vi "ZeroMQ Command Generator.vi"() -> ()   [LabVIEW 2018]
uses:
  <vilib>/addons/zeromq/socket_type.ctl
  <vilib>/addons/zeromq/socket_options.ctl
  <vilib>/addons/zeromq/zmq_context.lvclass
  <vilib>/addons/zeromq/zeromq.lvlib
  <vilib>/addons/zeromq/zmq_socket.lvclass
panel:
  out "reply":string
  in  "data":string="hello"
  in  "send":bool
  in  "reqEndpoint":string="tcp://200.131.64.126:54883"
  out "repMsg":string
  in  "repEndpoint":string="tcp://200.131.64.126:54032"
  in  "appendCR":bool caption="Append \n CR-LF"
  in  "pushAddress":string="tcp://200.131.64.170:54031" caption="PUSH address (=PUB+1, before start)"
  out "ledFocuser":bool
  out "ledWeather":bool
  out "ledTCSPD":bool
  out "ledS4ICS":bool
  in  "0mqPubAarray":string[](array[string])=["tcp://200.131.64.237:7001", "tcp://200.131.64.237:7005", "tcp://200.131.64.236:50350", "tcp://200.131.64.126:54030"] caption="Publisher Addresses"
  out "dataS4ICS":string caption="S4ICS"
  in  "stop":bool
  in  "push":bool caption="PUSH"
  in  "cmd in":string="{ \"clientId\": 666,  \"clientTransactionId\": 0,\n        \"clientName\": \"Simulator\", \"action\": \"STATUS\" }" caption="Message to send"
  out "dataFocuser":string caption="Focuser 160"
  out "dataMeteor":string caption="Estação Meteorológica"
  out "dataTCSPD":string caption="TCSPD"
  # "ZeroMQ Command Simulator - SUB & PUSH"
  # "Pedido de status para WheatherT160:"
  # "{ \"clientId\": 123, \"clientTransactionId\": 1234, \"clientName\": \"Simulator\", \"action\": \"STATUS\" }"
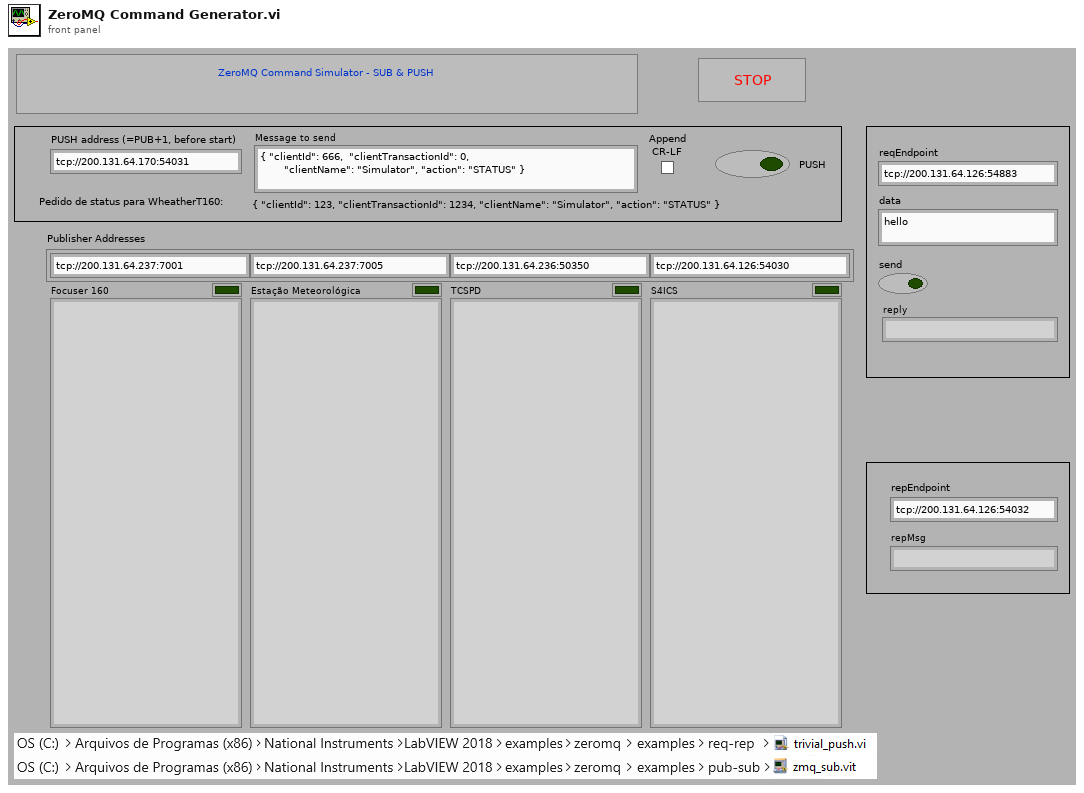
[diagram p1: front panel]
types:
  T1 = typedef "zeromq.lvlib/socket_type.ctl" = enum8{"ZMQ_PAIR", "ZMQ_PUB", "ZMQ_SUB", "ZMQ_REQ", "ZMQ_REP", "ZMQ_DEALER", "ZMQ_ROUTER", "ZMQ_PULL", "ZMQ_PUSH", "ZMQ_XPUB", "ZMQ_XSUB", "ZMQ_STREAM", "ZMQ_SERVER", "ZMQ_CLIENT", "ZMQ_RADIO", "ZMQ_DISH", "ZMQ_GATHER", "ZMQ_SCATTER", "ZMQ_DGRAM"}
  T2 = typedef "zeromq.lvlib/socket_options.ctl" = enum8{"NONE", "ZMQ_HWM", "<2>", "ZMQ_SWAP", "ZMQ_AFFINITY", "ZMQ_ROUTING_ID", "ZMQ_SUBSCRIBE", "ZMQ_UNSUBSCRIBE", "ZMQ_RATE", "ZMQ_RECOVERY_IVL", "ZMQ_MCAST_LOOP", "ZMQ_SNDBUF", "ZMQ_RCVBUF", "ZMQ_RCVMORE", "ZMQ_FD", "ZMQ_EVENTS", "ZMQ_TYPE", "ZMQ_LINGER", "ZMQ_RECONNECT_IVL", "ZMQ_BACKLOG", "ZMQ_RECOVERY_IVL_MSEC", "ZMQ_RECONNECT_IVL_MAX", "ZMQ_MAXMSGSIZE", "ZMQ_SNDHWM", "ZMQ_RCVHWM", "ZMQ_MULTICAST_HOPS", "<26>", "ZMQ_RCVTIMEO", "ZMQ_SNDTIMEO", "<29>", "<30>", "ZMQ_IPV4ONLY", "ZMQ_LAST_ENDPOINT", "ZMQ_ROUTER_MANDATORY", "ZMQ_TCP_KEEPALIVE", "ZMQ_TCP_KEEPALIVE_CNT", "ZMQ_TCP_KEEPALIVE_IDLE", "ZMQ_TCP_KEEPALIVE_INTVL", "ZMQ_TCP_ACCEPT_FILTER", "ZMQ_IMMEDIATE", "ZMQ_XPUB_VERBOSE", "ZMQ_ROUTER_RAW", "ZMQ_IPV6", "ZMQ_MECHANISM", "ZMQ_PLAIN_SERVER", "ZMQ_PLAIN_USERNAME", "ZMQ_PLAIN_PASSWORD", "ZMQ_CURVE_SERVER", "ZMQ_CURVE_PUBLICKEY", "ZMQ_CURVE_SECRETKEY", "ZMQ_CURVE_SERVERKEY", "ZMQ_PROBE_ROUTER", "ZMQ_REQ_CORRELATE", "ZMQ_REQ_RELAXED", "ZMQ_CONFLATE", "ZMQ_ZAP_DOMAIN", "ZMQ_ROUTER_HANDOVER", "ZMQ_TOS", "ZMQ_IPC_FILTER_PID", "ZMQ_IPC_FILTER_UID", "ZMQ_IPC_FILTER_GID", "ZMQ_CONNECT_ROUTING_ID", "ZMQ_GSSAPI_SERVER", "ZMQ_GSSAPI_PRINCIPAL", "ZMQ_GSSAPI_SERVICE_PRINCIPAL", "ZMQ_GSSAPI_PLAINTEXT", "ZMQ_HANDSHAKE_IVL", "<67>", "ZMQ_SOCKS_PROXY", "ZMQ_XPUB_NODROP", "ZMQ_BLOCKY", "ZMQ_XPUB_MANUAL", "ZMQ_XPUB_WELCOME_MSG", "ZMQ_STREAM_NOTIFY", "ZMQ_INVERT_MATCHING", "ZMQ_HEARTBEAT_IVL", "ZMQ_HEARTBEAT_TTL", "ZMQ_HEARTBEAT_TIMEOUT", "ZMQ_XPUB_VERBOSER", "ZMQ_CONNECT_TIMEOUT", "ZMQ_TCP_MAXRT", "ZMQ_THREAD_SAFE", "<82>", "<83>", "ZMQ_MULTICAST_MAXTPDU", "ZMQ_VMCI_BUFFER_SIZE", "ZMQ_VMCI_BUFFER_MIN_SIZE", "ZMQ_VMCI_BUFFER_MAX_SIZE", "ZMQ_VMCI_CONNECT_TIMEOUT", "ZMQ_USE_FD", "ZMQ_GSSAPI_PRINCIPAL_NAMETYPE", "ZMQ_GSSAPI_SERVICE_PRINCIPAL_NAMETYPE", "ZMQ_BINDTODEVICE", "ZMQ_ZAP_ENFORCE_DOMAIN", "ZMQ_LOOPBACK_FASTPATH", "ZMQ_METADATA", "ZMQ_MULTICAST_LOOP", "ZMQ_ROUTER_NOTIFY"}
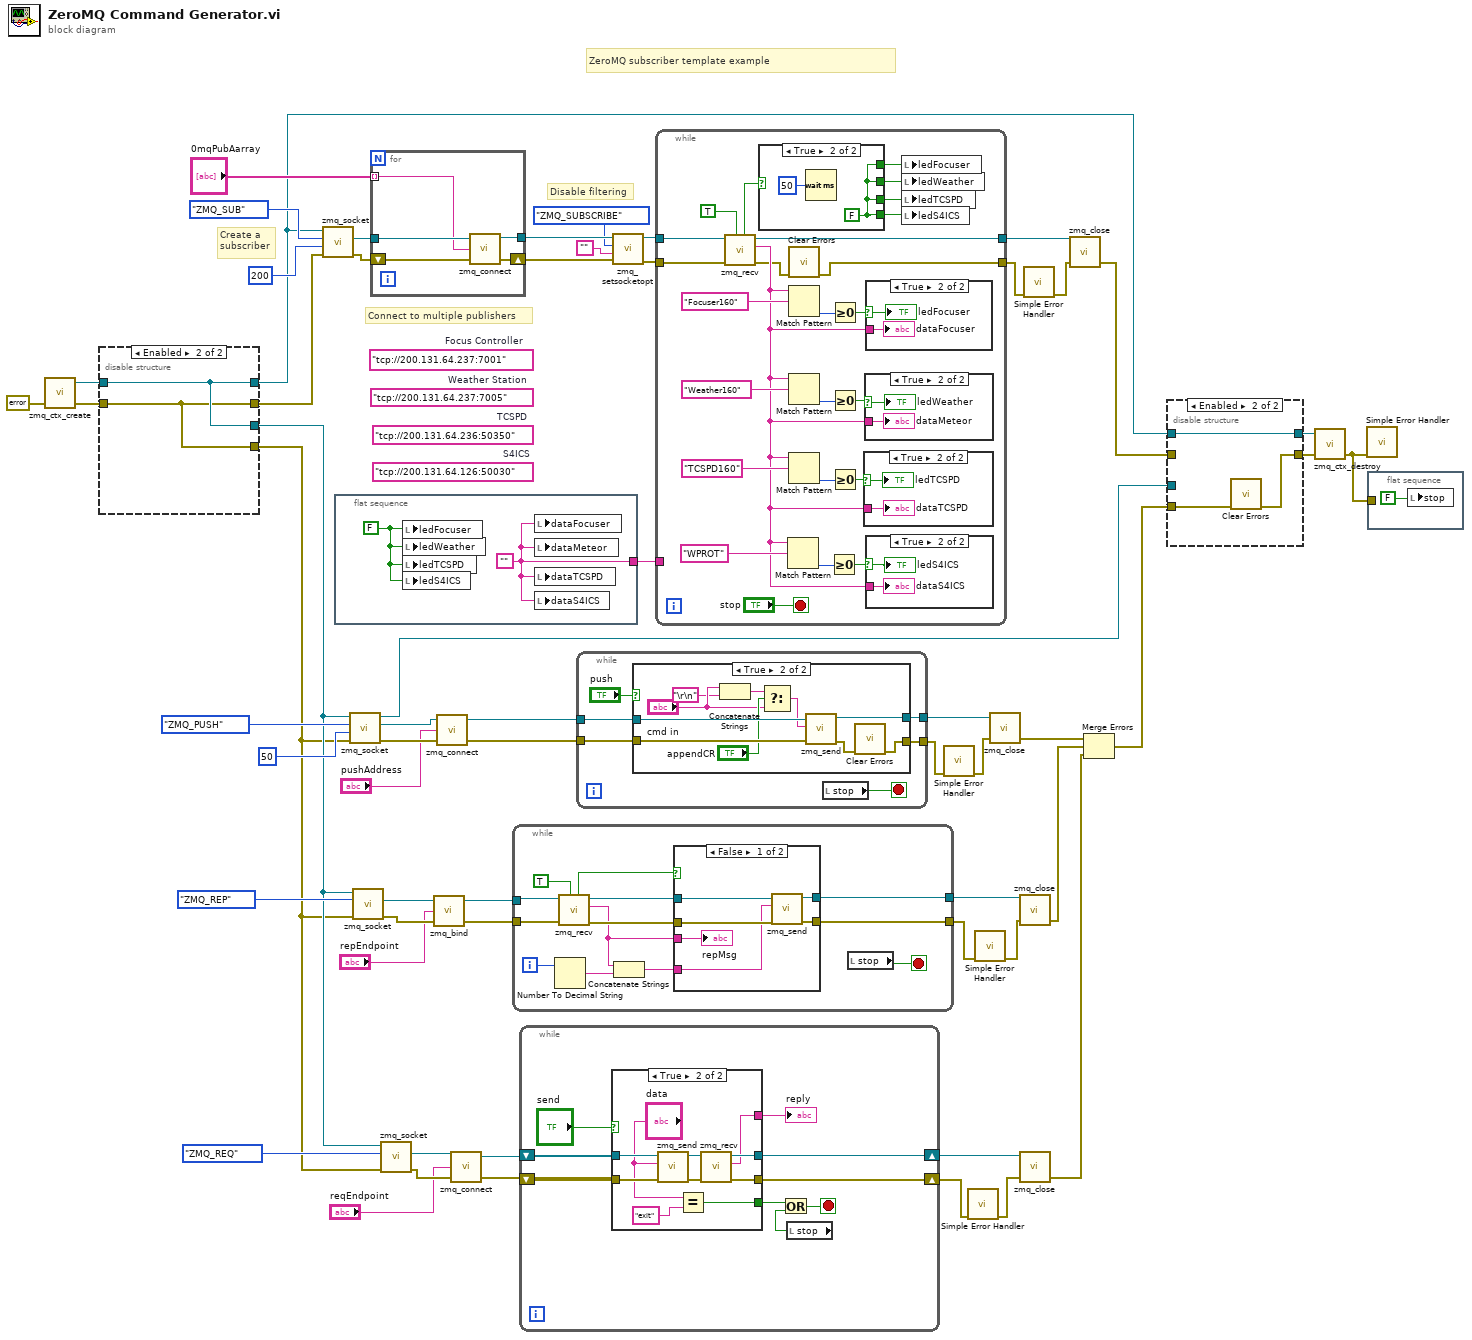
[diagram p0: block diagram]
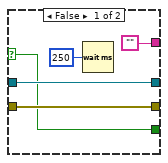
[diagram p2: hidden frame]
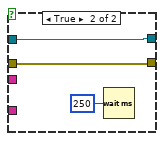
[diagram p3: hidden frame]
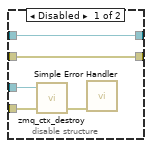
[diagram p4: hidden frame]
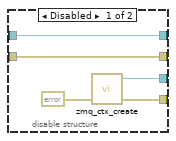
[diagram p5: hidden frame]
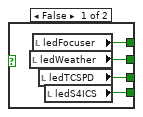
[diagram p7: hidden frame]
diagram:
  (unwired) "tcp://200.131.64.126:50030"  # S4ICS
  (unwired) "tcp://200.131.64.236:50350"  # TCSPD
  (unwired) "tcp://200.131.64.237:7005"  # Weather Station
  (unwired) "tcp://200.131.64.237:7001"  # Focus Controller
  # "ZeroMQ subscriber template example"
  # "Create a \nsubscriber"
  # "Disable filtering"
  # "Connect to multiple publishers"
  n1 = call <vilib>:"zmq_ctx_create.vi"("error in"=errorcluster {"status"=FALSE, "code"=0, "source"=""}) -> ("error out"=w32:errorcluster, "context out"=w31:refnum<class "zmq_context.lvclass">)  [unwired: 3 in]
  n2 = disable-structure shown="Enabled" {
    disable-tunnel: [w63 w66] -> w10
    disable-tunnel: [w62 w65] -> w9
    disable-tunnel: w32 -> [w60 w65]
    disable-tunnel: w31 -> [w61 w66]
    disable-tunnel: [w61 w66] -> w29
    disable-tunnel: [w60 w65] -> w30
    frame Disabled {
      n3 = call <vilib>:"zmq_ctx_create.vi"("error in"=errorcluster {"status"=FALSE, "code"=0, "source"=""}) -> ("error out"=w62:errorcluster, "context out"=w63:refnum<class "zmq_context.lvclass">)  [unwired: 3 in]
    }
    frame Enabled {
    }
  }
  n4 = call <vilib>:"zmq_socket.vi"("error in"=w30, "linger (ms)"=200, "socket type"=socket_type."ZMQ_SUB", "context in"=w29) -> ("error out"=w58:errorcluster, "socket out"=w51:refnum<class "zmq_socket.lvclass">)  [unwired: 1 in, 1 out]
  n5 = flat-sequence {
    tunnel: [w68] -> w39
    frame #0 {
      w67 = FALSE
      w68 = ""
      n6 = local write "ledFocuser"(w67) -> ()
      n7 = local write "ledWeather"(w67) -> ()
      n8 = local write "ledTCSPD"(w67) -> ()
      n9 = local write "ledS4ICS"(w67) -> ()
      n10 = local write "dataFocuser"(w68) -> ()
      n11 = local write "dataMeteor"(w68) -> ()
      n12 = local write "dataTCSPD"(w68) -> ()
      n13 = local write "dataS4ICS"(w68) -> ()
    }
  }
  n14 = call <vilib>:"zmq_socket.vi"("error in"=w9, "linger (ms)"=50, "socket type"=socket_type."ZMQ_PUSH", "context in"=w10) -> ("error out"=w47:errorcluster, "socket out"=w46:refnum<class "zmq_socket.lvclass">, "context out"=w37:refnum<class "zmq_context.lvclass">)  [unwired: 1 in]
  n15 = call <vilib>:"zmq_socket.vi"("error in"=w9, "socket type"=socket_type."ZMQ_REP", "context in"=w10) -> ("error out"=w23:errorcluster, "socket out"=w24:refnum<class "zmq_socket.lvclass">)  [unwired: 2 in, 1 out]
  n16 = for {
    tunnel: w51 -> [w73]
    tunnel: [w71] -> w57
    shift-right: [w70] -> w56
    shift-left: w58 -> [w72]
    tunnel: "0mqPubAarray" -> [w69] mode=indexing
    n17 = call <vilib>:"zmq_connect.vi"("error in"=w72, "endpoint"=w69, "socket in"=w73) -> ("error out"=w70:errorcluster, "socket out"=w71:refnum<class "zmq_socket.lvclass">)  [unwired: 1 in]
  }
  n18 = call <vilib>:"zmq_socket.vi"("error in"=w9, "socket type"=socket_type."ZMQ_REQ", "context in"=w10) -> ("error out"=w17:errorcluster, "socket out"=w16:refnum<class "zmq_socket.lvclass">)  [unwired: 2 in, 1 out]
  n19 = call <vilib>:"zmq_bind.vi"("error in"=w23, "endpoint"="repEndpoint", "socket in"=w24) -> ("error out"=w19:errorcluster, "socket out"=w20:refnum<class "zmq_socket.lvclass">)  [unwired: 1 in]
  n20 = call <vilib>:"zmq_connect.vi"("error in"=w47, "endpoint"="pushAddress", "socket in"=w46) -> ("error out"=w44:errorcluster, "socket out"=w45:refnum<class "zmq_socket.lvclass">)  [unwired: 1 in]
  n21 = call <vilib>:"zmq_connect.vi"("error in"=w17, "endpoint"="reqEndpoint", "socket in"=w16) -> ("error out"=w15:errorcluster, "socket out"=w14:refnum<class "zmq_socket.lvclass">)  [unwired: 1 in]
  n22 = while {
    tunnel: w20 -> [w85]
    tunnel: w19 -> [w86]
    tunnel: [w78] -> w8
    tunnel: [w82] -> w21
    i -> [w81]
    stop <- w74 stop-if-true
    n23 = Number To Decimal String(number=w81) -> (decimal integer string=w80:string)  [unwired: 1 in]
    n24 = call <vilib>:"zmq_recv.vi"("no block? (F)"=TRUE, "error in"=w86, "socket in"=w85) -> ("error out"=w84:errorcluster, "data"=w75:string, "socket out"=w83:refnum<class "zmq_socket.lvclass">, "timeout?"=w76:bool)  [unwired: 2 in, 1 out]
    n25 = Concatenate Strings(w75, w80) -> (w79:string)
    n26 = case shown="False" w76 {
      tunnel: w84 -> [w92 w94]
      tunnel: w83 -> [w91 w95]
      tunnel: [w90 w95] -> w82
      tunnel: w79 -> [w89 _]
      tunnel: [w88 w94] -> w78
      tunnel: w75 -> [w87 _]
      frame False {
        n27 = call <vilib>:"zmq_send.vi"("error in"=w92, "data"=w89, "socket in"=w91) -> ("error out"=w88:errorcluster, "socket out"=w90:refnum<class "zmq_socket.lvclass">)  [unwired: 4 in]
        "repMsg" <- w87
      }
      frame True {
        n28 = Wait (ms)(milliseconds to wait=u32 250) -> ()  [unwired: 1 out]
      }
    }
    n29 = local read "stop"() -> (w74:bool)
  }
  n30 = while {
    shift-right: [w102] -> w5
    shift-left: w15 -> [w104]
    shift-right: [w101] -> w13
    shift-left: w14 -> [w103]
    stop <- w99 stop-if-true
    n31 = case shown="True" "send" {
      selector: "send" -> [w106 _]
      tunnel: w104 -> [w108 w119]
      tunnel: w103 -> [w109 w118]
      tunnel: [w108 w116] -> w102
      tunnel: [w109 w115] -> w101
      tunnel: [w106 w111] -> w98
      tunnel: ["" w110] -> w96
      frame False {
        n32 = Wait (ms)(milliseconds to wait=u32 250) -> ()  [unwired: 1 out]
      }
      frame True {
        n33 = call <vilib>:"zmq_send.vi"("error in"=w119, "data"="data", "socket in"=w118) -> ("error out"=w114:errorcluster, "socket out"=w117:refnum<class "zmq_socket.lvclass">)  [unwired: 4 in]
        n34 = Equal?(x="data", y="exit") -> (x = y?=w111:bool)
        n35 = call <vilib>:"zmq_recv.vi"("error in"=w114, "socket in"=w117) -> ("error out"=w116:errorcluster, "data"=w110:string, "socket out"=w115:refnum<class "zmq_socket.lvclass">)  [unwired: 3 in, 2 out]
      }
    }
    "reply" <- w96
    n36 = local read "stop"() -> (w97:bool)
    n37 = Or(x=w98, y=w97) -> (x .or. y?=w99:bool)
  }
  n38 = while {
    tunnel: w45 -> [w125]
    tunnel: w44 -> [w124]
    tunnel: [w122] -> w43
    tunnel: [w120] -> w35
    stop <- w121 stop-if-true
    n39 = case shown="True" "push" {
      tunnel: w125 -> [w126 w137]
      tunnel: w124 -> [w127 w136]
      tunnel: [w126 w135] -> w122
      tunnel: [w127 w128] -> w120
      frame False {
      }
      frame True {
        n40 = Concatenate Strings("cmd in", "\r\n") -> (w133:string)
        n41 = Select(t=w133, s="appendCR", f="cmd in") -> (s? t:f=w134:string)
        n42 = call <vilib>:"zmq_send.vi"("error in"=w136, "data"=w134, "socket in"=w137) -> ("error out"=w129:errorcluster, "socket out"=w135:refnum<class "zmq_socket.lvclass">)  [unwired: 4 in]
        n43 = call <vilib>:"Clear Errors.vi"("error in (no error)"=w129) -> ("error out"=w128:errorcluster)  [unwired: 5 in, 1 out]
      }
    }
    n44 = local read "stop"() -> (w121:bool)
  }
  n45 = call <vilib>:"zmq_setsocketopt.vi"("error in"=w56, "value"="", "option"=socket_options."ZMQ_SUBSCRIBE", "socket in"=w57) -> ("error out"=w55:errorcluster, "socket out"=w54:refnum<class "zmq_socket.lvclass">)  [unwired: 2 in]
  n46 = while {
    tunnel: w54 -> [w162]
    tunnel: w55 -> [w161]
    tunnel: [w138] -> w36
    tunnel: [w151] -> w50
    tunnel: w39 -> [_]
    stop <- "stop" stop-if-true
    n47 = call <vilib>:"zmq_recv.vi"("no block? (F)"=TRUE, "error in"=w161, "socket in"=w162) -> ("error out"=w139:errorcluster, "data"=w145:string, "socket out"=w151:refnum<class "zmq_socket.lvclass">, "timeout?"=w144:bool)  [unwired: 2 in, 1 out]
    n48 = case shown="True" w144 {
      tunnel: [w166 w167] -> w143
      tunnel: [w165 w167] -> w142
      tunnel: [w164 w167] -> w141
      tunnel: [w163 w167] -> w140
      frame False {
        n49 = local read "ledWeather"() -> (w164:bool)
        n50 = local read "ledFocuser"() -> (w165:bool)
        n51 = local read "ledTCSPD"() -> (w163:bool)
        n52 = local read "ledS4ICS"() -> (w166:bool)
      }
      frame True {
        w167 = FALSE
        n53 = Wait (ms)(milliseconds to wait=u32 50) -> ()  [unwired: 1 out]
      }
    }
    n54 = Match Pattern(string=w145, regular expression="WPROT") -> (offset past match=w150:i32)  [unwired: 1 in, 3 out]
    n55 = call <vilib>:"Clear Errors.vi"("error in (no error)"=w139) -> ("error out"=w138:errorcluster)  [unwired: 5 in, 1 out]
    n56 = Match Pattern(string=w145, regular expression="Focuser160") -> (offset past match=w158:i32)  [unwired: 1 in, 3 out]
    n57 = Match Pattern(string=w145, regular expression="Weather160") -> (offset past match=w160:i32)  [unwired: 1 in, 3 out]
    n58 = Match Pattern(string=w145, regular expression="TCSPD160") -> (offset past match=w156:i32)  [unwired: 1 in, 3 out]
    n59 = Greater Or Equal To 0?(x=w150) -> (x >= 0?=w149:bool)
    n60 = Greater Or Equal To 0?(x=w158) -> (x >= 0?=w157:bool)
    n61 = Greater Or Equal To 0?(x=w160) -> (x >= 0?=w159:bool)
    n62 = Greater Or Equal To 0?(x=w156) -> (x >= 0?=w155:bool)
    n63 = case shown="True" w155 {
      selector: w155 -> [_ w175]
      tunnel: w145 -> [_ w176]
      frame False {
      }
      frame True {
        "dataTCSPD" <- w176
        "ledTCSPD" <- w175
      }
    }
    n64 = case shown="True" w159 {
      selector: w159 -> [_ w173]
      tunnel: w145 -> [_ w174]
      frame False {
      }
      frame True {
        "dataMeteor" <- w174
        "ledWeather" <- w173
      }
    }
    n65 = case shown="True" w157 {
      selector: w157 -> [_ w171]
      tunnel: w145 -> [_ w172]
      frame False {
      }
      frame True {
        "dataFocuser" <- w172
        "ledFocuser" <- w171
      }
    }
    n66 = case shown="True" w149 {
      selector: w149 -> [_ w169]
      tunnel: w145 -> [_ w170]
      frame False {
      }
      frame True {
        "dataS4ICS" <- w170
        "ledS4ICS" <- w169
      }
    }
    n67 = local write "ledFocuser"(w142) -> ()
    n68 = local write "ledWeather"(w141) -> ()
    n69 = local write "ledTCSPD"(w140) -> ()
    n70 = local write "ledS4ICS"(w143) -> ()
  }
  n71 = call <vilib>:"Simple Error Handler.vi"("error in (no error)"=w35) -> ("error out"=w34:errorcluster)  [unwired: 4 in, 4 out]
  n72 = call <vilib>:"Simple Error Handler.vi"("error in (no error)"=w5) -> ("error out"=w6:errorcluster)  [unwired: 4 in, 4 out]
  n73 = call <vilib>:"Simple Error Handler.vi"("error in (no error)"=w8) -> ("error out"=w7:errorcluster)  [unwired: 4 in, 4 out]
  n74 = call <vilib>:"zmq_close.vi"("error in"=w34, "socket"=w43) -> ("error out"=w4:errorcluster)  [unwired: 3 in]
  n75 = call <vilib>:"zmq_close.vi"("error in"=w7, "socket"=w21) -> ("error out"=w3:errorcluster)  [unwired: 3 in]
  n76 = call <vilib>:"zmq_close.vi"("error in"=w6, "socket"=w13) -> ("error out"=w2:errorcluster)  [unwired: 3 in]
  n77 = call <vilib>:"Simple Error Handler.vi"("error in (no error)"=w36) -> ("error out"=w33:errorcluster)  [unwired: 4 in, 4 out]
  n78 = call <vilib>:"zmq_close.vi"("error in"=w33, "socket"=w50) -> ("error out"=w28:errorcluster)  [unwired: 3 in]
  n79 = Merge Errors(w4, w3, w2) -> (w1:errorcluster)
  n80 = disable-structure shown="Enabled" {
    disable-tunnel: w37 -> [w180 _]
    disable-tunnel: w1 -> [w179 w182]
    disable-tunnel: w29 -> [w177 w184]
    disable-tunnel: w28 -> [w178 _]
    disable-tunnel: [w178 w183] -> w27
    disable-tunnel: [w177 w184] -> w26
    frame Disabled {
      n81 = call <vilib>:"zmq_ctx_destroy.vi"("error in"=w179, "context in"=w180) -> ("error out"=w181:errorcluster)  [unwired: 3 in]
      n82 = call <vilib>:"Simple Error Handler.vi"("error in (no error)"=w181) -> ()  [unwired: 4 in, 5 out]
    }
    frame Enabled {
      n83 = call <vilib>:"Clear Errors.vi"("error in (no error)"=w182) -> ("error out"=w183:errorcluster)  [unwired: 5 in, 1 out]
    }
  }
  n84 = call <vilib>:"zmq_ctx_destroy.vi"("error in"=w27, "context in"=w26) -> ("error out"=w18:errorcluster)  [unwired: 3 in]
  n85 = call <vilib>:"Simple Error Handler.vi"("error in (no error)"=w18) -> ()  [unwired: 4 in, 5 out]
  n86 = flat-sequence {
    tunnel: w18 -> [_]
    frame #0 {
      n87 = local write "stop"(FALSE) -> ()
    }
  }
